vi "All_Combined_final_opt_save_file_in_pc.vi"() -> ()   [LabVIEW 2018]
uses:
  <vilib>/LabVIEW Interface for Arduino/Type Defs/Board Type.ctl
  Controls created/Control 3.ctl
  Controls created/Control 4.ctl
  <vilib>/LabVIEW Interface for Arduino/Type Defs/Connection Type.ctl
  <instrlib>/LeCroy Wave Series/Public/Data/Read Single Waveform.vi
  <vilib>/LabVIEW Interface for Arduino/LabVIEW Interface for Arduino.lvlib
  <instrlib>/Siglent SDG X Series/Siglent SDG X Series.lvlib
  <instrlib>/LeCroy Wave Series/LeCroy Wave Series.lvlib
panel:
  in  "Tab Control":enum32{"Page 1", "Page 2", "Page 3"}(tab)
  in  "VISA resource":refnum<visa-resource-name>
  in  "Board Type (Uno)":T1
  in  "Steps for 1 rotation(1600steps)":i16=1600
  in  "Set Speed (Steps/s)":i16=1200 min=0 max=3000 step=50
  out "Steps Remaining? 2":bool
  in  "Step Size":i16
  out "Step Angle":dbl
  in  "Baud Rate":u32=115200
  out "Iteration #":i32
  out "Steps Remaining?":bool
  in  "Total translation distance(in mm)":i16
  out "Error":errorcluster
  in  "Step size":dbl
  in  "Arbitray Movement":bool
  in  "Stop":bool
  out "Moving?":bool
  out "stop motion":bool
  in  "MOTION":bool
  in  "?":i8(slide) step=2 scale=0.0..2.0
  in  "OK Button":bool
  out "# steps moved":i32
  in  "VISA Refnum in":refnum<visa-resource-name>="USB0::0xF4EC::0xEE38::SDG2XCAD2R3765::INSTR"
  in  "Channel (1:Channel 1)":i32(ring)=1 items=["Channel 1"=1, "Channel 2"=2]
  in  "Enable Output (T: Enable)":bool=TRUE
  in  "Amplitude (1.0 Vpp)":dbl=20.0 format="%#.3f"
  in  "Frequency (1000 Hz)":T2=1500000.0 format="%#.6g"
  in  "DC Offset (0.00 V) in":dbl
  in  "Waveform Function (0: Sine) in":u16(ring) items=["Sine", "Square", "Ramp", "DC", "Pulse", "Arb"]
  in  "Phase (0.0 degrees)":dbl=0.002 min=-360.0 max=360.0 format="%#.1g"
  in  "Fall (20 ns)":dbl=8.4e-09 format="%#.3g"
  in  "Duty (20%)":dbl=4.32 min=0.0001 max=100.0 format="%.4g"
  in  "Delay (0.00 s)":dbl min=-1000000.0 max=1000000.0
  in  "Rise (20 ns)":dbl=1.04e-08 format="%#.3g"
  in  "True To \ngenerate\n pulse":T3=TRUE
  out "VISA resource name out":refnum<visa-resource-name>
  out "error out":errorcluster
  out "Output Filename":path
  out "error out 2":errorcluster
  in  "format string":string="Channel: %g \nWavetype: %g \nAMP: %gV\nFreq: %gHz \nRiseTime: %gs \nFallTime: %gs \nDutyCycle: %g"
  out "Output Directory":path
  in  "File Directory":path=path "E:/Ankur/Labview/Automation/Data/Exp1"
  in  "Filename":string
  out "Oscilloscope\n Runnning":bool
  in  "stop":bool
  out "Waveform Data":waveform(dbl)(graph)
  in  "Timeout (10000 ms)":u32=10000
  in  "Source (0: Channel 1)":u16(ring) items=["Channel 1", "Channel 2", "Channel 3", "Channel 4", "Memory 1", "Memory 2", "Memory 3", "Memory 4", "Function 1", "Function 2", "Function 3", "Function 4", "Function 5", "Function 6", "Function 7", "Function 8"]
  in  "Perform Auto Setup?":bool
  in  "Reset Scope?":bool
  in  "VISA resource name":refnum<visa-resource-name>="LecroyHDO4024-1"
  in  "Save Files in Directory (In Oscilloscope)":string="D:\\Automation\\Data"
  in  "Filename":string="Title"
  in  "Path to save DATA":path=path "E:/Ankur/Labview/Automation/Files/Oscdata"
  out "Saved filename":string
  in  "Save File locally":bool
  # "For Rotational motion"
  # "For Translational Motion"
  # "For Translational motion"
  # "OFF"
  # "ON"
  # "Yes"
  # "No"
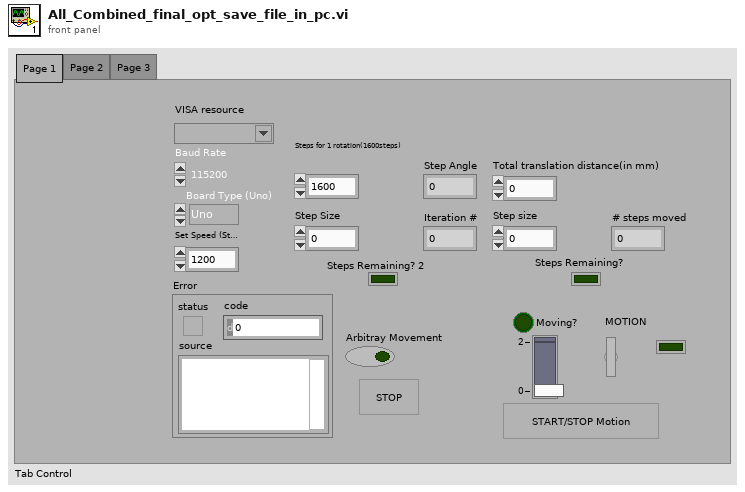
[diagram p1: front panel]
types:
  T1 = typedef "LabVIEW Interface for Arduino.lvlib/Board Type.ctl" = enum16{"Uno", "Dimuelanove w/Atmega 328", "Mega 2560"}
  T2 = typedef "Control 3.ctl" = dbl
  T3 = typedef "Control 4.ctl" = bool
  T4 = typedef "LabVIEW Interface for Arduino.lvlib/Connection Type.ctl" = enum8{"USB / Serial", "XBEE", "BlueSmirf (Bluetooth)"}
  T5 = typedef "LabVIEW Interface for Arduino.lvlib/Arduino Resource.ctl" = cluster{"VISA resource":refnum<visa-resource-name>, "Board Type":T1, "Connection Type":enum8{"USB / Serial"}, "Bytes Per Packet (15)":u8}
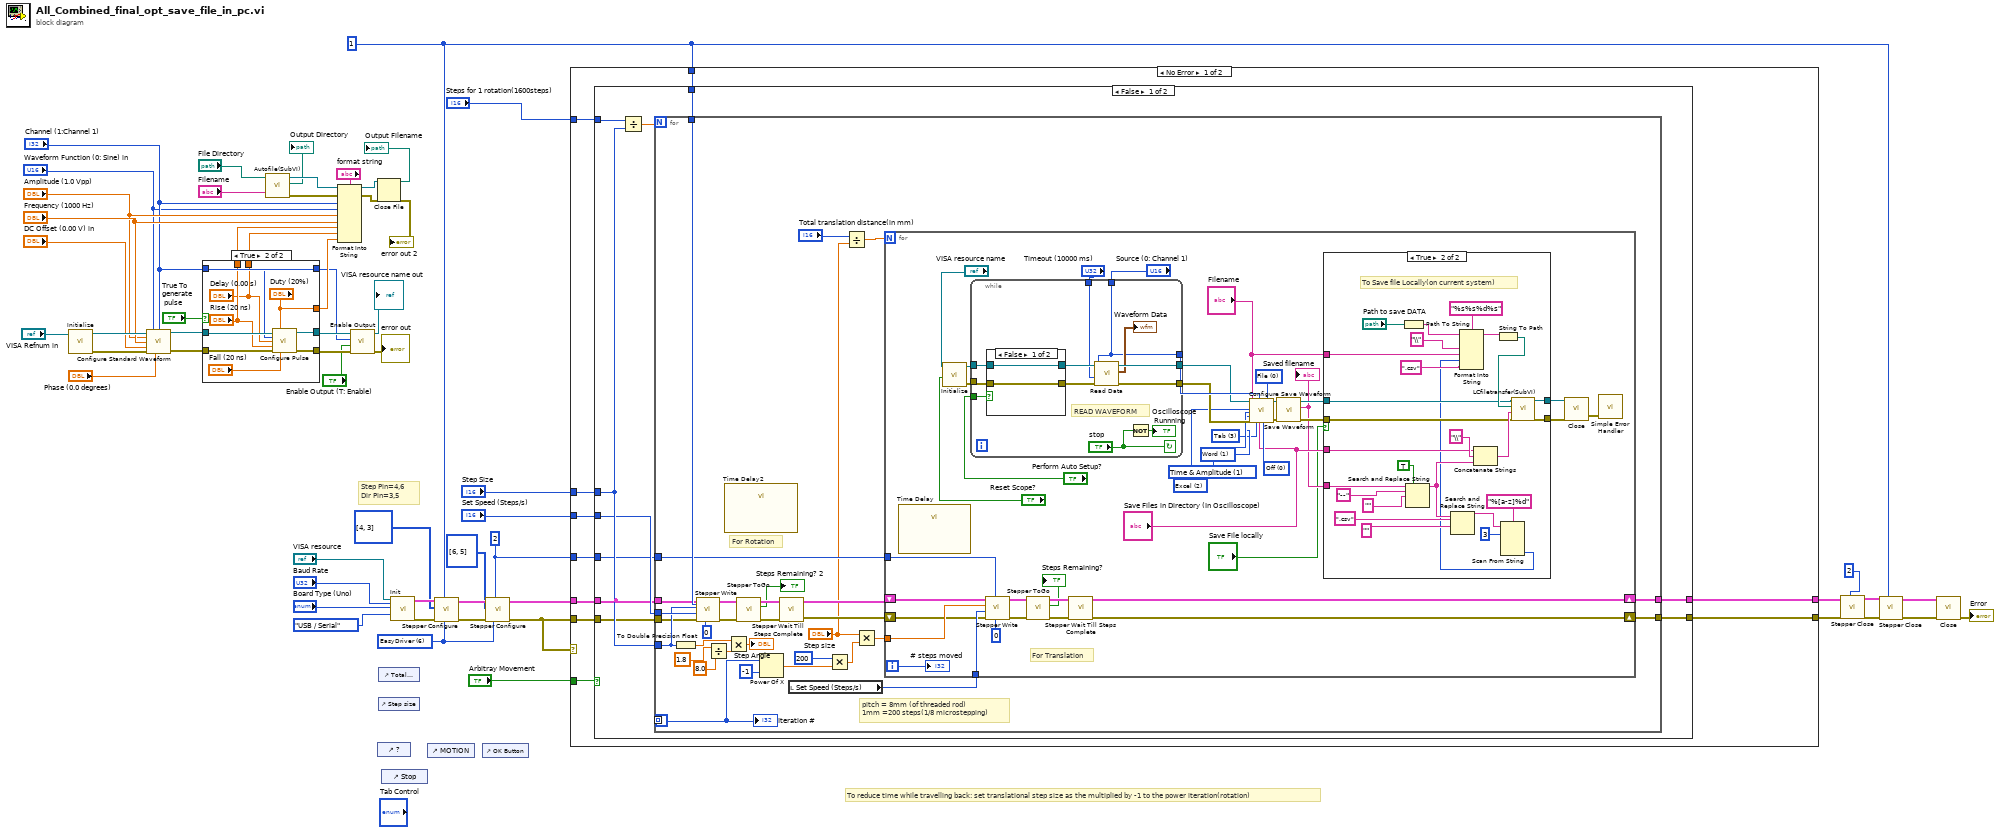
[diagram p0: block diagram]
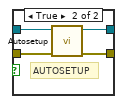
[diagram p3: hidden frame]
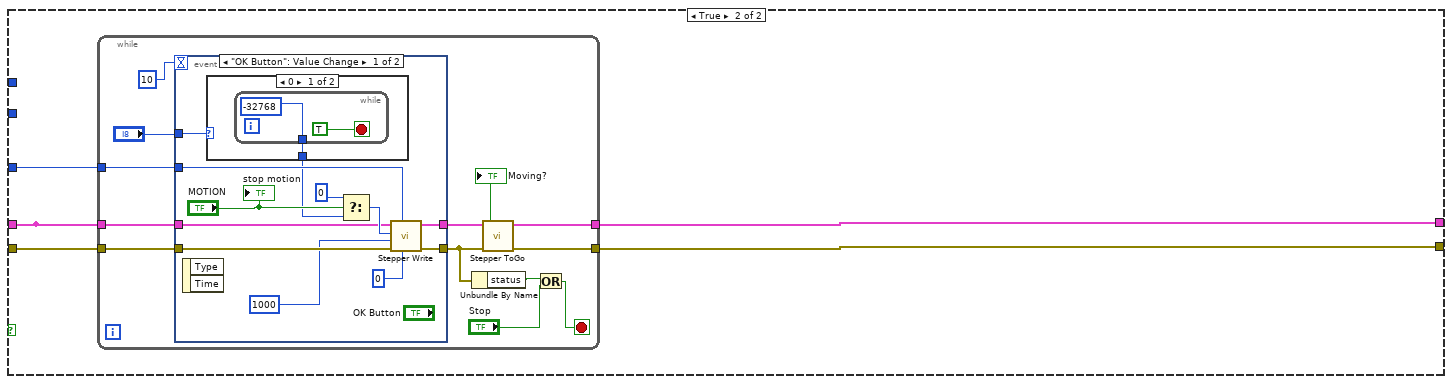
[diagram p4: hidden frame]
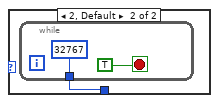
[diagram p5: hidden frame]
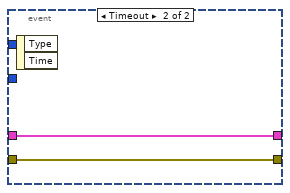
[diagram p6: hidden frame]
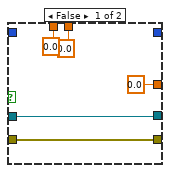
[diagram p8: hidden frame]
diagram:
  w41 = u8 2 ("Stepper #")
  w10 = u8 1 ("Stepper #")
  w42 = u8 6 items=["2 Wire (Pulse & Direction)"=1, "2 Wire"=2, "4 Wire"=4, "EasyDriver"=6, "AF Motor Shield (Stepper 1 & 2 Only)"=5] ("Control Method")
  # "To reduce time while travelling back: set translational step size as the multiplied by -1 to the power iteration(rotation)"
  # "Step Pin=4,6\nDir Pin=3,5"
  n1 = call <instrlib>:"Initialize.vi"("VISA resource name"="VISA Refnum in") -> ("error out"=w35:errorcluster, "VISA resource name out"=w36:refnum<visa-resource-name>)  [unwired: 9 in]
  n2 = call <instrlib>:"Configure Standard Waveform.vi"("VISA resource name"=w36, "Waveform Function (0: Sine)"="Waveform Function (0: Sine) in", "Channel (1:Channel 1)"="Channel (1:Channel 1)", "Amplitude (1.0 Vpp)"="Amplitude (1.0 Vpp)", "Frequency (1000 Hz)"="Frequency (1000 Hz)", "DC Offset (0.00 V)"="DC Offset (0.00 V) in", "error in (no error)"=w35, "Phase (0.0 degrees)"="Phase (0.0 degrees)") -> ("VISA resource name out"=w31:refnum<visa-resource-name>, "error out"=w34:errorcluster)  [unwired: 6 in]
  n3 = case shown="True" "True To \ngenerate\n pulse" {
    tunnel: [w62 w70] -> w40
    tunnel: [w61 w69] -> w39
    tunnel: w31 -> [w62 w68]
    tunnel: w34 -> [w61 w67]
    tunnel: "Channel (1:Channel 1)" -> [_ w66]
    tunnel: "Channel (1:Channel 1)" -> [_ _]
    tunnel: [0.0 ("Duty (20%)") "Duty (20%)"] -> w27
    tunnel: [0.0 ("Rise (20 ns)") "Rise (20 ns)"] -> w19
    tunnel: [0.0 ("Delay (0.00 s)") "Delay (0.00 s)"] -> w18
    frame False {
    }
    frame True {
      n4 = call <instrlib>:"Configure Pulse.vi"("VISA resource name"=w68, "Duty (20%)"="Duty (20%)", "Channel (1:Channel 1)"=w66, "Delay (0.00 s)"="Delay (0.00 s)", "Rise (20 ns)"="Rise (20 ns)", "error in (no error)"=w67, "Fall (20 ns)"="Fall (20 ns)") -> ("VISA resource name out"=w70:refnum<visa-resource-name>, "error out"=w69:errorcluster)  [unwired: 7 in]
    }
  }
  n5 = call "Autofile(SubVI).vi"("Filename"="Filename", "File Directory"="File Directory") -> ("error out"=w14:errorcluster, "Output Directory"=→"Output Directory":path, "Byte Stream File out"=w15:refnum<file>)  [unwired: 7 in]
  n6 = Format Into String(format string="format string", initial string=w15, error in=w14, "Channel (1:Channel 1)", "Waveform Function (0: Sine) in", "Amplitude (1.0 Vpp)", "Frequency (1000 Hz)", w19, w18, w27) -> (resulting string=w26:refnum<file>, error out=w23:errorcluster)
  n7 = call <instrlib>:"Enable Output.vi"("error in (no error)"=w39, "Enable Output (T: Enable)"="Enable Output (T: Enable)", "Channel (1:Channel 1)"="Channel (1:Channel 1)", "VISA resource name"=w40) -> ("error out"=→"error out":errorcluster, "VISA resource name out"=→"VISA resource name out":refnum<visa-resource-name>)  [unwired: 6 in]
  n8 = Close File(refnum=w26, error in=w23) -> (path=→"Output Filename":path, error out=→"error out 2":errorcluster)
  n9 = control-ref of="?"() -> ()  [unwired: 1 out]
  n10 = control-ref of="Total translation distance(in mm)"() -> ()  [unwired: 1 out]
  n11 = control-ref of="Step size"() -> ()  [unwired: 1 out]
  n12 = control-ref of="Stop"() -> ()  [unwired: 1 out]
  n13 = call <vilib>:"Init.vi"("VISA resource"="VISA resource", "Baud Rate (115200)"="Baud Rate", "Board Type (Uno)"="Board Type (Uno)", "Connection Type (USB/Serial)"=Connection_Type."USB / Serial") -> ("Arduino Resource"=w54:T5, "error out"=w53:errorcluster)  [unwired: 14 in]
  n14 = control-ref of="MOTION"() -> ()  [unwired: 1 out]
  n15 = call <vilib>:"Stepper Configure.vi"("Control Method"=w42, "Stepper #"=w10, "error in"=w53, "Stepper Pins"=u8[] [4, 3], "Arduino Resource"=w54) -> ("error out"=w44:errorcluster, "Arduino Resource Out"=w45:T5)  [unwired: 5 in]
  n16 = control-ref of="OK Button"() -> ()  [unwired: 1 out]
  n17 = call <vilib>:"Stepper Configure.vi"("Control Method"=w42, "Stepper #"=w41, "error in"=w44, "Stepper Pins"=u8[] [6, 5], "Arduino Resource"=w45) -> ("error out"=w6:errorcluster, "Arduino Resource Out"=w7:T5)  [unwired: 5 in]
  n18 = case shown="No Error" w6 {
    tunnel: [w75 w249] -> w2
    tunnel: [w82 w250] -> w1
    tunnel: [w81 w250] -> _
    tunnel: "Step Size" -> [w80 _]
    tunnel: "Steps for 1 rotation(1600steps)" -> [w79 _]
    tunnel: "Set Speed (Steps/s)" -> [w78 _]
    tunnel: "Arbitray Movement" -> [w77 _]
    tunnel: w10 -> [w76 _]
    tunnel: w41 -> [w74 _]
    tunnel: w7 -> [w73 w250]
    tunnel: w6 -> [w72 w249]
    frame No Error {
      n19 = case shown="False" w77 {
        tunnel: [w91 w215] -> w82
        tunnel: [w84 w213] -> w81
        tunnel: w80 -> [w89 _]
        tunnel: w79 -> [w88 _]
        tunnel: w78 -> [w87 _]
        tunnel: w76 -> [w86 _]
        tunnel: [w92 w211] -> w75
        tunnel: w74 -> [w85 w214]
        tunnel: w73 -> [w84 w213]
        tunnel: w72 -> [w83 w212]
        frame False {
          n20 = Divide(x=w88, y=w89) -> (x/y=w90:dbl)
          n21 = for {
            N: w90 -> [_]
            tunnel: [w93] -> w92
            tunnel: [w94] -> w91
            tunnel: w87 -> [w120]
            tunnel: [w100] -> _ mode=indexing
            tunnel: w89 -> [w115]
            tunnel: w86 -> [w110]
            tunnel: w85 -> [w109]
            tunnel: w84 -> [w102]
            tunnel: w83 -> [w101]
            i -> [w100]
            # "pitch = 8mm (of threaded rod)\n1mm =200 steps(1/8 microstepping)"
            # "For Rotation"
            n22 = To Double Precision Float(number=w115) -> (double precision float=w116:dbl)
            n23 = call <vilib>:"Stepper Write.vi"("Set Acceleration (0 to disable)"=i16 0 ("Acceleration"), "Stepper #"=w110, "error in"=w101, "Set Speed (Steps per Second)"=w120, "# of Steps to Move"=w115, "Arduino Resource"=w102) -> ("error out"=w119:errorcluster, "Arduino Resource Out"=w118:T5)  [unwired: 4 in]
            n24 = Divide(x=1.8 ("y"), y=8.0) -> (x/y=w105:dbl)
            n25 = call "Time Delay2"() -> ()  [unwired: 11 in, 1 out]
            n26 = Multiply(x=w116, y=w105) -> (x*y=→"Step Angle":dbl)
            n27 = call <vilib>:"Stepper ToGo.vi"("error in"=w119, "Arduino Resource"=w118) -> ("error out"=w123:errorcluster, "Steps Remaining?"=→"Steps Remaining? 2":bool, "Arduino Resource Out"=w122:T5)  [unwired: 6 in, 1 out]
            n28 = Power Of X(1:-1 ("x"), 2:w100) -> (0:w95:dbl)
            n29 = call <vilib>:"Stepper Wait Till Steps Complete.vi"("error in"=w123, "Arduino Resource In"=w122) -> ("error out"=w114:errorcluster, "Arduino Resource Out"=w113:T5)  [unwired: 8 in]
            n30 = local read "Set Speed (Steps/s)"() -> (w112:i16)
            n31 = Multiply(x=i16 200 ("y"), y=w95) -> (x*y=w97:dbl)
            n32 = Divide(x="Total translation distance(in mm)", y="Step size") -> (x/y=w103:dbl)
            n33 = Multiply(x="Step size", y=w97) -> (x*y=w107:dbl)
            n34 = for {
              N: w103 -> [_]
              shift-right: [w159] -> w94
              shift-left: w113 -> [w155]
              shift-right: [w158] -> w93
              shift-left: w114 -> [w154]
              tunnel: w107 -> [w157]
              tunnel: w112 -> [w156]
              tunnel: w109 -> [w151]
              i -> [w152]
              w137 = u16 3 items=["Comma", "Space", "Semicolon", "Tab"] ("Delimiter (  0:Comma)")
              w136 = u16 0 items=["Off", "Wrap", "Fill"] ("Auto Save (0:Off")
              w138 = u16 1 items=["Byte", "Word", "Auto"] ("BinarySubFormat (1: Word)")
              w139 = u16 1 items=["Amplitude Only", "Time & Amplitude", "With Header"] ("SubFormat (1: Time & Amplitude)")
              w140 = u16 2 items=["Binary", "ASCII", "Excel", "MATLAB", "MathCad", "WaveML"] ("Format (0: Binary)")
              w135 = u16 0 items=["File", "M1", "M2", "M3", "M4"] ("Destination (0:File)")
              # "For Translation"
              n35 = call "Time Delay"() -> ()  [unwired: 11 in, 1 out]
              n36 = call <instrlib>:"Initialize.vi"("Reset? (T: Yes)"="Reset Scope?", "VISA resource name"="VISA resource name") -> ("error out"=w143:errorcluster, "VISA resource name out"=w142:refnum<visa-resource-name>)  [unwired: 8 in]
              n37 = while {
                tunnel: [w202] -> w149
                tunnel: [w201] -> w148
                tunnel: "Perform Auto Setup?" -> [w200]
                tunnel: "Source (0: Channel 1)" -> [w193]
                tunnel: w143 -> [w199]
                tunnel: w142 -> [w198]
                tunnel: "Timeout (10000 ms)" -> [w197]
                tunnel: [w193] -> w150
                stop <- "stop" continue-if-true
                # "READ WAVEFORM"
                n38 = case shown="False" w200 {
                  tunnel: w199 -> [w205 w210]
                  tunnel: w198 -> [w206 w209]
                  tunnel: [w206 w208] -> w204
                  tunnel: [w205 w207] -> w203
                  frame False {
                  }
                  frame True {
                    # "AUTOSETUP"
                    n39 = call <instrlib>:"Autosetup.vi"("error in (no error)"=w210, "VISA resource name"=w209) -> ("error out"=w207:errorcluster, "VISA resource name out"=w208:refnum<visa-resource-name>)  [unwired: 8 in]
                  }
                }
                n40 = call-poly <instrlib>:"Read Data.vi"("error in (no error)"=w203, "Timeout (10000 ms)"=w197, "Source (0: Channel 1)"=w193, "VISA resource name"=w204) -> ("error out"=w202:errorcluster, "Waveform Data"=→"Waveform Data":waveform(dbl), "VISA resource name out"=w201:refnum<visa-resource-name>)  [unwired: 5 in]
                n41 = Not(x="stop") -> (.not. x?=→"Oscilloscope\n Runnning":bool)
              }
              n42 = call <vilib>:"Stepper Write.vi"("Set Acceleration (0 to disable)"=i16 0, "Stepper #"=w151, "error in"=w154, "Set Speed (Steps per Second)"=w156, "# of Steps to Move"=w157, "Arduino Resource"=w155) -> ("error out"=w161:errorcluster, "Arduino Resource Out"=w160:T5)  [unwired: 4 in]
              n43 = call <vilib>:"Stepper ToGo.vi"("error in"=w161, "Arduino Resource"=w160) -> ("error out"=w164:errorcluster, "Steps Remaining?"=→"Steps Remaining?":bool, "Arduino Resource Out"=w163:T5)  [unwired: 6 in, 1 out]
              n44 = call <vilib>:"Stepper Wait Till Steps Complete.vi"("error in"=w164, "Arduino Resource In"=w163) -> ("error out"=w158:errorcluster, "Arduino Resource Out"=w159:T5)  [unwired: 8 in]
              n45 = call <instrlib>:"Configure Save Waveform.vi"("VISA resource name"=w148, "Trace Title (Title)"="Filename", "Format (0: Binary)"=w140, "SubFormat (1: Time & Amplitude)"=w139, "BinarySubFormat (1: Word)"=w138, "error in (no error)"=w149, "Delimiter (  0:Comma)"=w137, "Source (0: Channel 1)"=w150, "Save Files in Directory (D:\\Waveforms)"="Save Files in Directory (In Oscilloscope)", "Auto Save (0:Off"=w136, "Destination (0:File)"=w135) -> ("VISA resource name out"=w134:refnum<visa-resource-name>, "error out"=w133:errorcluster)  [unwired: 7 in]
              n46 = call <instrlib>:"Save Waveform.vi"("error in (no error)"=w133, "VISA resource name"=w134) -> ("error out"=w128:errorcluster, "Saved filename"=w126:string, "VISA resource name out"=w127:refnum<visa-resource-name>)  [unwired: 7 in]
              "Saved filename" <- w126
              n47 = case shown="True" "Save File locally" {
                tunnel: [w166 w189] -> w131
                tunnel: [w165 w188] -> w130
                tunnel: "Save Files in Directory (In Oscilloscope)" -> [_ w182]
                tunnel: w128 -> [w165 w181]
                tunnel: w127 -> [w166 w180]
                tunnel: w126 -> [_ w179]
                tunnel: "Filename" -> [_ w178]
                frame False {
                }
                frame True {
                  # "To Save file Locally(on current system)"
                  n48 = Path To String(path="Path to save DATA") -> (string=w183:string)
                  n49 = Search and Replace String(replace all?=TRUE ("replace all? (F)"), input string=w179, search string="--", replace string="" ("replace string (\"\")")) -> (result string=w174:string)  [unwired: 4 in, 3 out]
                  n50 = Search and Replace String(input string=w174, search string=".csv", replace string="" ("replace string (\"\")")) -> (result string=w177:string)  [unwired: 5 in, 3 out]
                  n51 = Concatenate Strings(w182, "\\" ("string"), w174) -> (w190:string)
                  n52 = Scan From String(format string="%[a-z]%d", input string=w177, initial scan location=u32 3) -> (output 2=w170:i32)  [unwired: 4 in, 3 out]
                  n53 = Format Into String(format string="%s%s%d%s", initial string=w183, "\\" ("input 1"), w178, w170, ".csv" ("input 3")) -> (resulting string=w169:string)  [unwired: 1 in, 1 out]
                  n54 = String To Path(string=w169) -> (path=w187:path)
                  n55 = call <userlib>:"LCfiletransfer(SubVI).vi"("error in (no error)"=w181, "Source Filename"=w190, "file path (use dialog)"=w187, "VISA Refnum in"=w180) -> ("error out"=w188:errorcluster, "VISA Refnum out"=w189:refnum<visa-resource-name>)  [unwired: 5 in, 1 out]
                }
              }
              n56 = call <vilib>:"Close.vi"("error in (no error)"=w130, "VISA resource name"=w131) -> ("error out"=w132:errorcluster)  [unwired: 9 in]
              n57 = call <vilib>:"Simple Error Handler.vi"("error in (no error)"=w132) -> ()  [unwired: 4 in, 5 out]
              "# steps moved" <- w152
            }
            "Iteration #" <- w100
          }
        }
        frame True {
          n58 = while {
            tunnel: [w221] -> w215
            tunnel: w214 -> [w220]
            tunnel: w213 -> [w218]
            tunnel: w212 -> [w217]
            tunnel: [w216] -> w211
            stop <- w227 stop-if-true
            n59 = event shown="[0] \"OK Button\": Value Change" {
              selector: _ -> [_ _]
              dyn-events: _ -> [_ _]
              timeout: 10 -> [_ _]
              tunnel: [w239 w248] -> w225
              tunnel: [w240 w247] -> w223
              tunnel: w220 -> [w235 _]
              tunnel: "?" -> [w234 _]
              tunnel: w218 -> [w231 w248]
              tunnel: w217 -> [w230 w247]
              event "OK Button": Value Change {
                n60 = event-data() -> ()  [unwired: 1 in, 2 out]
                n61 = case shown="0" w234 {
                  tunnel: [w241 w244] -> w232
                  frame 0 {
                    n62 = while {
                      tunnel: [i16 -32768 ("# of Steps to Move")] -> w241
                      stop <- TRUE ("Stop Reverse movement") stop-if-true
                    }
                  }
                  frame 2, Default {
                    n63 = while {
                      tunnel: [i16 32767 ("# of Steps to Move")] -> w244
                      stop <- TRUE ("Stop Forward movement") stop-if-true
                    }
                  }
                }
                n64 = Select(t=0, s="MOTION", f=w232) -> (s? t:f=w236:i32)
                n65 = call <vilib>:"Stepper Write.vi"("Set Acceleration (0 to disable)"=i16 0 ("Set acceleration"), "Stepper #"=w235, "error in"=w230, "Set Speed (Steps per Second)"=i16 1000, "# of Steps to Move"=w236, "Arduino Resource"=w231) -> ("error out"=w240:errorcluster, "Arduino Resource Out"=w239:T5)  [unwired: 4 in]
                "stop motion" <- "MOTION"
              }
              event Timeout {
                n66 = event-data() -> ()  [unwired: 1 in, 2 out]
              }
            }
            n67 = Unbundle By Name(w223) -> ("status"=w226:bool)
            n68 = call <vilib>:"Stepper ToGo.vi"("error in"=w223, "Arduino Resource"=w225) -> ("error out"=w216:errorcluster, "Steps Remaining?"=→"Moving?":bool, "Arduino Resource Out"=w221:T5)  [unwired: 6 in, 1 out]
            n69 = Or(x=w226, y="Stop") -> (x .or. y?=w227:bool)
          }
        }
      }
    }
    frame Error {
    }
  }
  n70 = call <vilib>:"Stepper Close.vi"("Stepper #"=u8 2, "error in"=w2, "Arduino Resource"=w1) -> ("error out"=w5:errorcluster, "Arduino Resource Out"=w4:T5)  [unwired: 7 in]
  n71 = call <vilib>:"Stepper Close.vi"("Stepper #"=w10, "error in"=w5, "Arduino Resource"=w4) -> ("error out"=w9:errorcluster, "Arduino Resource Out"=w8:T5)  [unwired: 7 in]
  n72 = call <vilib>:"Close.vi"("Arduino Resource"=w8, "error in"=w9) -> ("error out"=→"Error":errorcluster)  [unwired: 13 in]
